vi "Snapshot Example.vi"() -> ()   [LabVIEW 2020]
uses:
  g_industrial_cam/Camera/Camera.lvclass/Camera.ctl
  g_industrial_cam/Buffer/Buffer.lvclass/Buffer.ctl
  g_industrial_cam/Buffer/Read Data as Mono10 Image.vi
  g_industrial_cam/Buffer/Read Data as Mono12 Image.vi
  g_industrial_cam/Buffer/Read Data as Mono14 Image.vi
  g_industrial_cam/Buffer/Read Data as Mono16 Image.vi
  g_industrial_cam/Camera/GetSetPixelFormat.vi
  g_industrial_cam/Buffer/Create from Handle.vi
  g_industrial_cam/Buffer/ReadDataAsMono2Byte.vi
  g_industrial_cam/Camera/Check Not Disconnected.vi
  g_industrial_cam/Buffer/Buffer.lvclass
  g_industrial_cam/Camera/Camera.lvclass
panel:
  in  "Take Snapshot":bool
  out "Timeout":bool
  out "Count":i32 caption="Snap Shot Count"
  out "Intensity Graph":u16[][](graph)
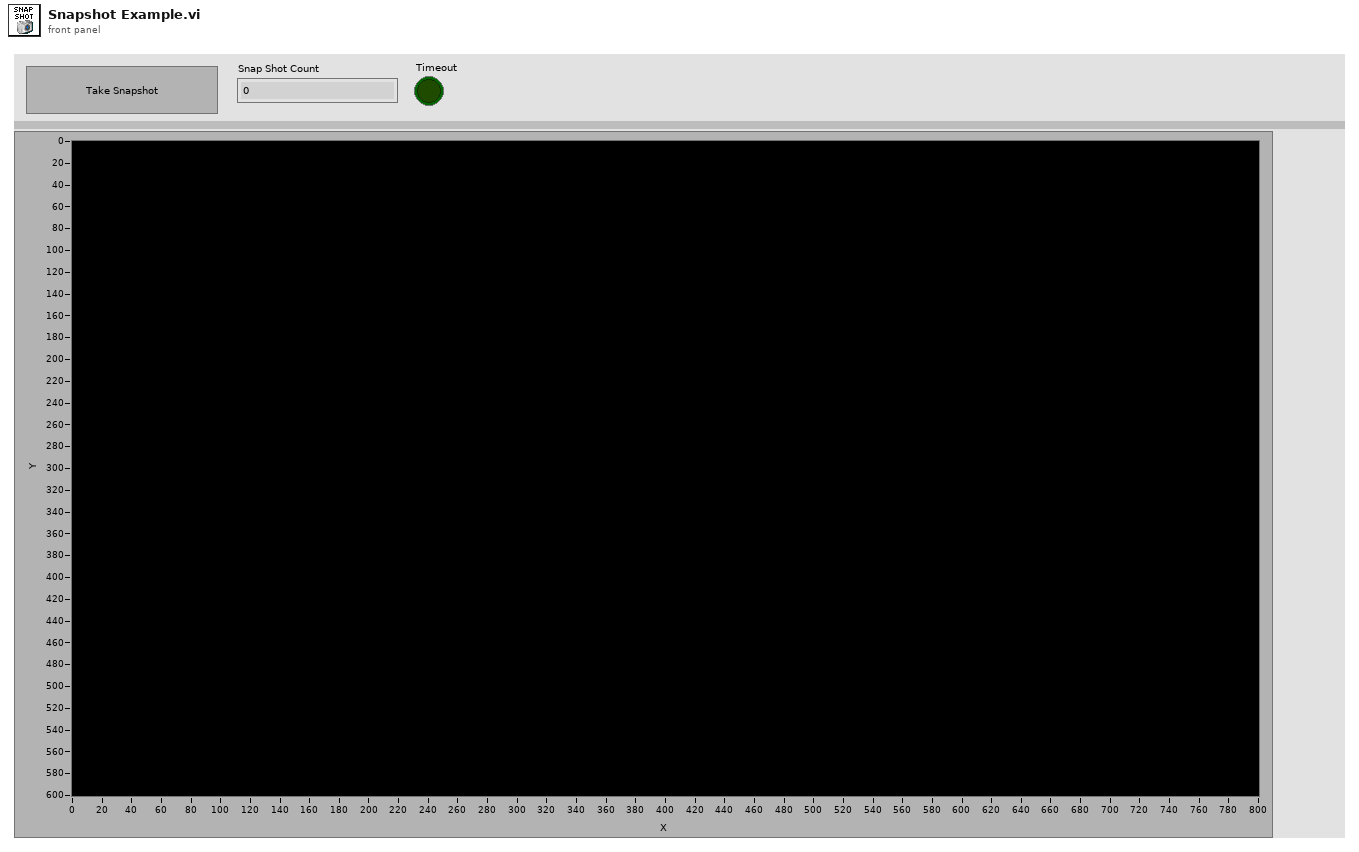
[diagram p1: front panel]
types:
  T1 = typedef "Device Enumeration.ctl" = cluster{"ID":string, "Protocol":string, "Vendor":string, "Model":string, "Serial":string, "Address":string}
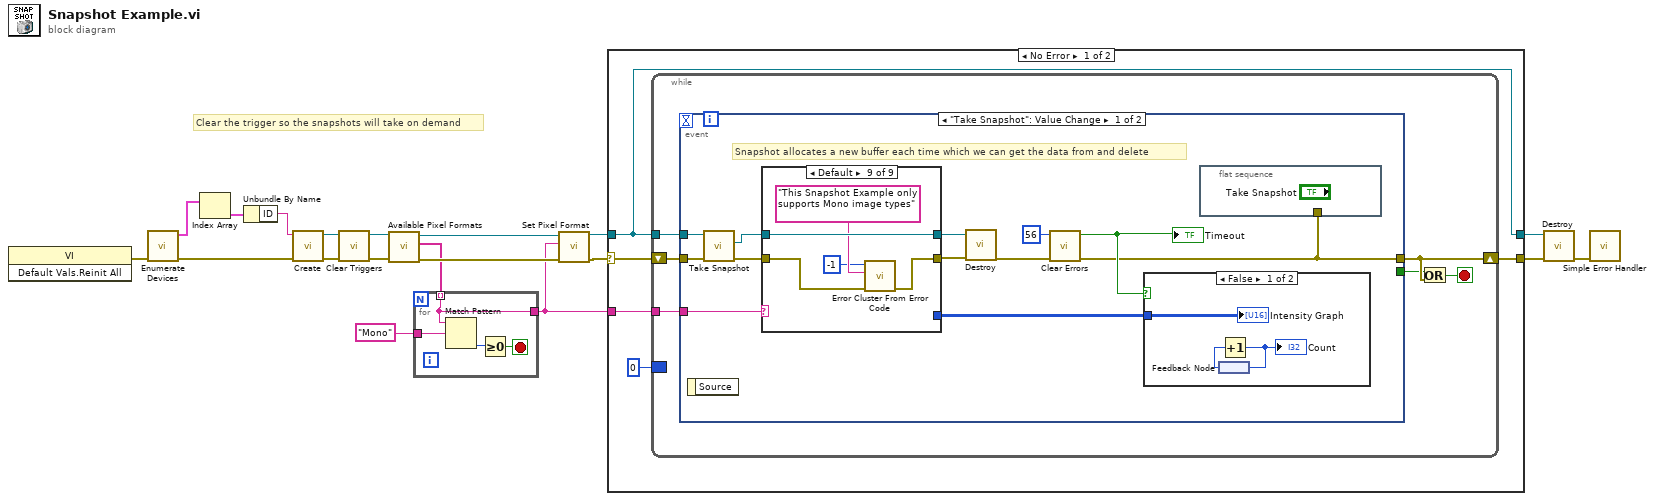
[diagram p0: block diagram]
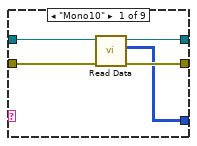
[diagram p2: hidden frame]
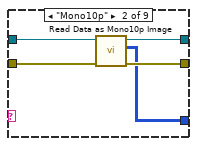
[diagram p3: hidden frame]
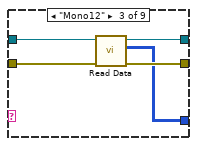
[diagram p4: hidden frame]
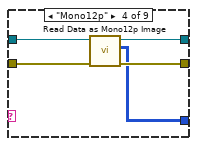
[diagram p5: hidden frame]
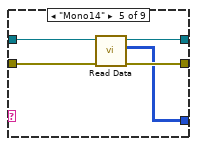
[diagram p6: hidden frame]
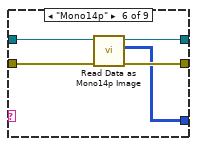
[diagram p7: hidden frame]
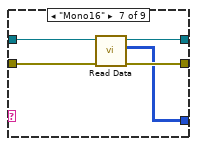
[diagram p8: hidden frame]
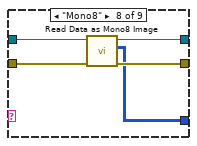
[diagram p9: hidden frame]
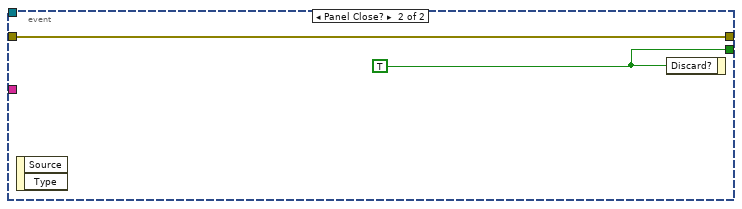
[diagram p11: hidden frame]
diagram:
  # "Clear the trigger so the snapshots will take on demand"
  n1 = invoke class="VI" method="Default Vals.Reinit All"() -> (error out=w4:errorcluster)  [unwired: 3 in, 2 out]
  n2 = call "Enumerate Devices.vi"("error in (no error)"=w4) -> ("error out"=w17:errorcluster, "Devices"=w19:T1[])  [unwired: 9 in]
  n3 = Index Array(array=w19) -> (element=w18:T1)  [unwired: 1 in]
  n4 = Unbundle By Name(w18) -> ("ID"=w16:string)
  n5 = call "Create.vi"("error in (no error)"=w17, "Identifier (ID, IP etc)"=w16) -> ("error out"=w15:errorcluster, "Camera"=w13:refnum<class "Camera.lvclass">)  [unwired: 8 in]
  n6 = call "Clear Triggers.vi"("error in (no error)"=w15, "Camera in"=w13) -> ("error out"=w9:errorcluster, "Camera"=w10:refnum<class "Camera.lvclass">)  [unwired: 8 in]
  n7 = call "Available Pixel Formats.vi"("error in (no error)"=w9, "Camera in"=w10) -> ("error out"=w6:errorcluster, "Pixel Formats"=w3:string[], "Camera"=w8:refnum<class "Camera.lvclass">)  [unwired: 7 in]
  n8 = for {
    tunnel: w3 -> [w23] mode=indexing
    tunnel: [w23] -> w1
    tunnel: "Mono" ("regular expression") -> [w20]
    stop <- w21 stop-if-true
    n9 = Match Pattern(string=w23, regular expression=w20) -> (offset past match=w22:i32)  [unwired: 1 in, 3 out]
    n10 = Greater Or Equal To 0?(x=w22) -> (x >= 0?=w21:bool)
  }
  n11 = call "Set Pixel Format.vi"("error in (no error)"=w6, "Pixel Format"=w1, "Camera in"=w8) -> ("error out"=w5:errorcluster, "Camera"=w7:refnum<class "Camera.lvclass">)  [unwired: 7 in]
  n12 = case shown="No Error" w5 {
    selector: w5 -> [w28 w97]
    tunnel: w7 -> [w26 w98]
    tunnel: [w27 w97] -> w12
    tunnel: [w26 w98] -> w14
    tunnel: w1 -> [w24 _]
    frame No Error {
      n13 = while {
        shift-right: [w31] -> w27
        shift-left: w28 -> [w33]
        tunnel: w26 -> [w34]
        border: 0 -> [_]
        tunnel: w24 -> [w29]
        stop <- w32 stop-if-true
        n14 = event shown="[0] \"Take Snapshot\": Value Change" {
          selector: _ -> [_ _]
          dyn-events: _ -> [_ _]
          timeout: _ -> [_ _]
          tunnel: w34 -> [w46 _]
          tunnel: w33 -> [w45 w96]
          tunnel: [w35 w96] -> w31
          tunnel: [_ w95] -> w30
          tunnel: w29 -> [w36 _]
          event "Take Snapshot": Value Change {
            # "Snapshot allocates a new buffer each time which we can get the data from and delete"
            n15 = event-data() -> ()  [unwired: 1 in, 1 out]
            n16 = call "Take Snapshot.vi"("error in (no error)"=w45, "Camera in"=w46) -> ("error out"=w40:errorcluster, "New Buffer"=w42:refnum<class "Buffer.lvclass">)  [unwired: 7 in, 1 out]
            n17 = case shown="Default" w36 {
              tunnel: [w47 w52 w57 w62 w67 w72 w77 w82 _] -> w43
              tunnel: w42 -> [w50 w56 w60 w66 w70 w76 w80 w86 w91]
              tunnel: [w48 w53 w58 w63 w68 w74 w78 w85 w91] -> w41
              tunnel: w40 -> [w49 w55 w59 w65 w69 w75 w79 w84 w89]
              tunnel: [w51 w54 w61 w64 w71 w73 w81 w83 w90] -> w38
              frame "Mono10" {
                n18 = call-poly "Read Data.vi"("error in (no error)"=w49, "Buffer in"=w50) -> ("error out"=w51:errorcluster, "Image"=w47:u16[][], "Buffer"=w48:refnum<class "Buffer.lvclass">)  [unwired: 7 in]
              }
              frame "Mono10p" {
                n19 = call "Read Data as Mono10p Image.vi"("error in (no error)"=w55, "Buffer in"=w56) -> ("error out"=w54:errorcluster, "Image"=w52:u16[][], "Buffer"=w53:refnum<class "Buffer.lvclass">)  [unwired: 7 in]
              }
              frame "Mono12" {
                n20 = call-poly "Read Data.vi"("error in (no error)"=w59, "Buffer in"=w60) -> ("error out"=w61:errorcluster, "Image"=w57:u16[][], "Buffer"=w58:refnum<class "Buffer.lvclass">)  [unwired: 7 in]
              }
              frame "Mono12p" {
                n21 = call "Read Data as Mono12p Image.vi"("error in (no error)"=w65, "Buffer in"=w66) -> ("error out"=w64:errorcluster, "Image"=w62:u16[][], "Buffer"=w63:refnum<class "Buffer.lvclass">)  [unwired: 7 in]
              }
              frame "Mono14" {
                n22 = call-poly "Read Data.vi"("error in (no error)"=w69, "Buffer in"=w70) -> ("error out"=w71:errorcluster, "Image"=w67:u16[][], "Buffer"=w68:refnum<class "Buffer.lvclass">)  [unwired: 7 in]
              }
              frame "Mono14p" {
                n23 = call "Read Data as Mono14p Image.vi"("error in (no error)"=w75, "Buffer in"=w76) -> ("error out"=w73:errorcluster, "Image"=w72:u16[][], "Buffer"=w74:refnum<class "Buffer.lvclass">)  [unwired: 7 in]
              }
              frame "Mono16" {
                n24 = call-poly "Read Data.vi"("error in (no error)"=w79, "Buffer in"=w80) -> ("error out"=w81:errorcluster, "Image"=w77:u16[][], "Buffer"=w78:refnum<class "Buffer.lvclass">)  [unwired: 7 in]
              }
              frame "Mono8" {
                n25 = call "Read Data as Mono8 Image.vi"("error in (no error)"=w84, "Buffer in"=w86) -> ("error out"=w83:errorcluster, "Image"=w82:u8[][], "Buffer"=w85:refnum<class "Buffer.lvclass">)  [unwired: 7 in]
              }
              frame Default {
                n26 = call <vilib>:"Error Cluster From Error Code.vi"("error in (no error)"=w89, "error message (\"\")"="This Snapshot Example only supports Mono image types" ("error message (\"\")"), "error code (0)"=-1) -> ("error out"=w90:errorcluster)  [unwired: 6 in]
              }
            }
            n27 = call "Destroy.vi"("error in (no error)"=w38, "Buffer in"=w41) -> ("error out"=w37:errorcluster)  [unwired: 9 in]
            n28 = call <vilib>:"Clear Errors.vi"("error in (no error)"=w37, "specific error code to clear (0: all)"=56) -> ("error out"=w35:errorcluster, "specific error cleared?"=w39:bool)  [unwired: 4 in]
            "Timeout" <- w39
            n29 = case shown="False" w39 {
              tunnel: w43 -> [w92 _]
              frame False {
                n30 = feedback #1() -> (w94:i32)
                n31 = Increment(x=w94) -> (x+1=w93:i32)
                "Count" <- w93
                n32 = feedback-in #1(w93) -> ()
                "Intensity Graph" <- w92
              }
              frame True {
              }
            }
            n33 = flat-sequence {
              tunnel: w35 -> [_]
              frame #0 {
              }
            }
          }
          event Panel Close? {
            w95 = TRUE
            n34 = event-data() -> ()  [unwired: 1 in, 2 out]
            n35 = event-data("Discard?"=w95) -> ()  [unwired: 1 in, 1 out]
          }
        }
        n36 = Or(x=w30, y=w31) -> (x .or. y?=w32:bool)
      }
    }
    frame Error {
    }
  }
  n37 = call "Destroy.vi"("error in (no error)"=w12, "Camera in"=w14) -> ("error out"=w11:errorcluster)  [unwired: 9 in]
  n38 = call <vilib>:"Simple Error Handler.vi"("error in (no error)"=w11) -> ()  [unwired: 4 in, 5 out]
